vi "Example Websockets ServerOnly.vi"() -> ()   [LabVIEW 2013]
uses:
  Connection.Websockets/Connection.WS.lvclass
  Connection/Connection.lvclass
panel:
  in  "remote port (8080)":u16=8080
  in  "Send":bool
  in  "String":string
  out "Received":string
  out "New connection":bool
  out "Client connected":bool
  out "listener error":errorcluster
  out "server session error":errorcluster
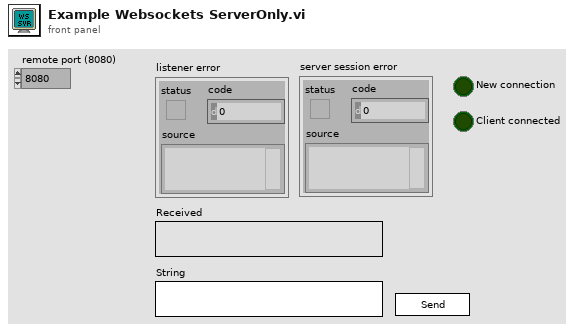
[diagram p1: front panel]
types:
  T1 = typedef "Connection.WS_GOSPL.lvlib/Connection.WS.lvclass/Websocket Frame Type -- ring.ctl" = u8
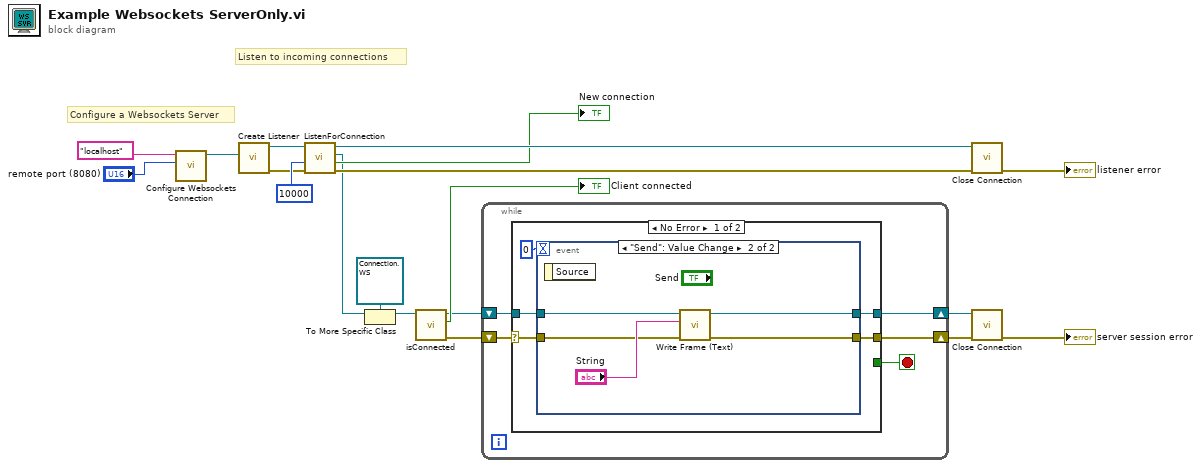
[diagram p0: block diagram]
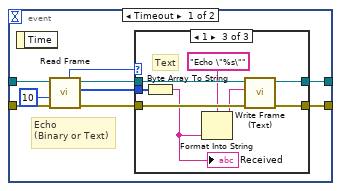
[diagram p2: hidden frame]
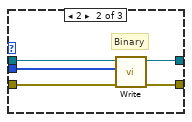
[diagram p4: hidden frame]
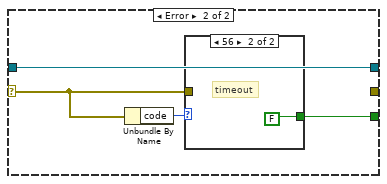
[diagram p5: hidden frame]
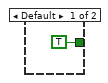
[diagram p6: hidden frame]
diagram:
  # "Listen to incoming connections"
  # "Configure a Websockets Server"
  n1 = call "Configure Websockets Connection.vi"("remote port (80)"="remote port (8080)", "address (localhost)"="localhost") -> ("Connection.Websockets"=w6:refnum<class "Connection.WS.lvclass">)  [unwired: 8 in, 1 out]
  n2 = call "Create Listener.vi"("Connection Configuration"=w6) -> ("error out"=w16:errorcluster, "Listener"=w19:refnum<class "Connection.WS.lvclass">)  [unwired: 9 in]
  n3 = call "ListenForConnection.vi"("error in (no error)"=w16, "timeout (2000 ms)"=10000 ("bytes to read (100)"), "Listener"=w19) -> ("error out"=w13:errorcluster, "New connection"=→"New connection":bool, "Connection"=w2:refnum<class "Connection.lvclass">, "Listener out"=w17:refnum<class "Connection.WS.lvclass">)  [unwired: 5 in]
  n4 = To More Specific Class(target class=refnum<class "Connection.WS.lvclass"> refnum ("Connection.WS"), reference=w2) -> (specific class reference=w7:refnum<class "Connection.WS.lvclass">)  [unwired: 1 in, 1 out]
  n5 = call "isConnected.vi"("Connection in"=w7) -> ("error out"=w4:errorcluster, "connected"=→"Client connected":bool, "Connection out"=w5:refnum<class "Connection.WS.lvclass">)  [unwired: 8 in]
  n6 = while {
    shift-right: [w24] -> w14
    shift-left: w5 -> [w23]
    shift-right: [w22] -> w1
    shift-left: w4 -> [w21]
    stop <- w20 stop-if-true
    n7 = case shown="No Error" w21 {
      selector: w21 -> [w26 w60]
      tunnel: [w29 w62] -> w24
      tunnel: w23 -> [w28 w62]
      tunnel: [w27 _] -> w22
      tunnel: [_ w59] -> w20
      frame No Error {
        n8 = event shown="[1] \"Send\": Value Change" {
          selector: _ -> [_ _]
          dyn-events: _ -> [_ _]
          timeout: 0 -> [_ _]
          tunnel: [w38 w54] -> w29
          tunnel: w28 -> [w37 w58]
          tunnel: [w31 w55] -> w27
          tunnel: w26 -> [w30 w56]
          event Timeout {
            # "Echo\n(Binary or Text)"
            n9 = event-data() -> ()  [unwired: 1 in, 1 out]
            n10 = call "Read Frame.vi"("error in (no error)"=w30, "timeout (1000 ms)"=10 ("bytes to read (100)"), "Connection.WS"=w37) -> ("error out"=w33:errorcluster, "Bytes"=w34:u8[], "Connection.WS"=w35:refnum<class "Connection.WS.lvclass">, "Frame Type"=w32:T1)  [unwired: 3 in, 2 out]
            n11 = case shown="1" w32 {
              tunnel: [w40 w45 w52] -> w38
              tunnel: [w39 w44 w51] -> w31
              tunnel: w35 -> [w40 w43 w53]
              tunnel: w34 -> [_ w42 w49]
              tunnel: w33 -> [w39 w41 w50]
              frame Default {
              }
              frame 2 {
                # "Binary"
                n12 = call "Write.vi"("error in (no error)"=w41, "Bytes"=w42, "Connection in"=w43) -> ("error out"=w44:errorcluster, "Connection"=w45:refnum<class "Connection.WS.lvclass">)  [unwired: 7 in]
              }
              frame 1 {
                # "Text"
                n13 = Byte Array To String(unsigned byte array=w49) -> (string=w48:string)
                "Received" <- w48
                n14 = Format Into String(format string="Echo \"%s\"", w48) -> (resulting string=w47:string)  [unwired: 2 in, 1 out]
                n15 = call "Write Frame (Text).vi"("error in (no error)"=w50, "Text"=w47, "Connection.WS"=w53) -> ("error out"=w51:errorcluster, "Connection.WS"=w52:refnum<class "Connection.WS.lvclass">)  [unwired: 7 in]
              }
            }
          }
          event "Send": Value Change {
            n16 = event-data() -> ()  [unwired: 1 in, 1 out]
            n17 = call "Write Frame (Text).vi"("error in (no error)"=w56, "Text"="String", "Connection.WS"=w58) -> ("error out"=w55:errorcluster, "Connection.WS"=w54:refnum<class "Connection.WS.lvclass">)  [unwired: 7 in]
          }
        }
      }
      frame Error {
        n18 = Unbundle By Name(w60) -> ("code"=w61:i32)
        n19 = case shown="56" w61 {
          tunnel: w60 -> [_ _]
          tunnel: [TRUE FALSE] -> w59
          frame Default {
          }
          frame 56 {
            # "timeout"
          }
        }
      }
    }
  }
  n20 = call "Close Connection.vi"("error in (no error)"=w13, "Connection in"=w17) -> ("error out"=→"listener error":errorcluster)  [unwired: 8 in, 1 out]
  n21 = call "Close Connection.vi"("error in (no error)"=w1, "Connection in"=w14) -> ("error out"=→"server session error":errorcluster)  [unwired: 8 in, 1 out]
